vi "PH_USB600x_AnalogReader.ProcEvents.vi"(0 "i ref in":refnum<vi>, 5 "error in":errorcluster) -> (14 "i ref out":refnum<vi>, 19 "error out":errorcluster)   [LabVIEW 2014, in "PH_USB600x_AnalogReader.lvlib"]
doc: "This method is used to define the events the object will listen to. Add your own events here."
uses:
  PH_USB600x_AnalogReader.lvlib
  CSCore/BaseProcess/BaseProcess.event definition.ctl
  CSCore/CAEObj/CAEObj.event definition.ctl
  CSCore/BaseProcess/BaseProcess.descriptor string definition.ctl
  CSCore/BaseProcess/BaseProcess.lvlib
  CSCore/CAEObj/CAEObj.lvlib
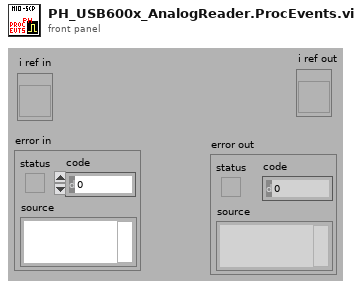
[diagram p1: front panel]
types:
  T1 = typedef "BaseProcess.lvlib/BaseProcess.event definition.ctl" = cluster{"CAEEvtDef":T2, "Data Descriptor":T3}
  T2 = typedef "CAEObj.lvlib/CAEObj.event definition.ctl" = cluster{"URL":string, "enable":bool, "ignoreResID":bool}
  T3 = typedef "BaseProcess.lvlib/BaseProcess.descriptor string definition.ctl" = string
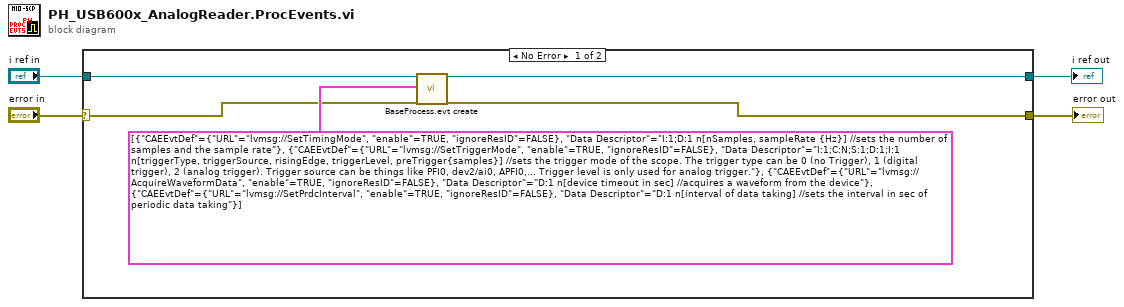
[diagram p0: block diagram]
diagram:
  n1 = case shown="No Error" "error in" {
    selector: "error in" -> [w5 w10]
    tunnel: "i ref in" -> [w9 w11]
    tunnel: [w7 w11] -> w3
    tunnel: [w6 w10] -> w2
    frame No Error {
      n2 = call "BaseProcess.evt create.vi"("i ref in"=w9, "newEvents"=T1[] [{"CAEEvtDef"={"URL"="lvmsg://SetTimingMode", "enable"=TRUE, "ignoreResID"=FALSE}, "Data Descriptor"="I:1;D:1 n[nSamples, sampleRate {Hz}] //sets the number of samples and the sample rate"}, {"CAEEvtDef"={"URL"="lvmsg://SetTriggerMode", "enable"=TRUE, "ignoreResID"=FALSE}, "Data Descriptor"="I:1;C:N;S:1;D:1;I:1 n[triggerType, triggerSource, risingEdge, triggerLevel, preTrigger{samples}] //sets the trigger mode of the scope. The trigger type can be 0 (no Trigger), 1 (digital trigger), 2 (analog trigger). Trigger source can be things like PFI0, dev2/ai0, APFI0,... Trigger level is only used for analog trigger."}, {"CAEEvtDef"={"URL"="lvmsg://AcquireWaveformData", "enable"=TRUE, "ignoreResID"=FALSE}, "Data Descriptor"="D:1 n[device timeout in sec] //acquires a waveform from the device"}, {"CAEEvtDef"={"URL"="lvmsg://SetPrdcInterval", "enable"=TRUE, "ignoreResID"=FALSE}, "Data Descriptor"="D:1 n[interval of data taking] //sets the interval in sec of periodic data taking"}] ("new events"), "error in (no error)"=w5) -> ("i ref out"=w7:refnum<vi>, "error out"=w6:errorcluster)  [unwired: 13 in, 2 out]
    }
    frame Error {
    }
  }
  "i ref out" <- w3
  "error out" <- w2
